vi "Lamp Name.vi"(7 "DB Data":variant[][](array[variant])) -> (1 "Led Name":string[](array[string]), 3 "Model Name":string)   [LabVIEW 2015]
uses:
  <vilib>/addons/database/_DB Variant To Data/Database Variant To Data.xnode
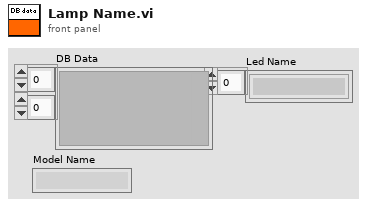
[diagram p1: front panel]
types:
  T1 = cluster{"Model Name":string, "Power Min":dbl, "Power Max":dbl, "Current Min":dbl, "Current Max":dbl, "Sleep Min ":dbl, "Sleep Max":dbl, "R-L Min":dbl, "R-L Max":dbl, "L-R Min":dbl, "L-R Max":dbl, "N-L Min":dbl, "N-L Max":dbl, "N-D Min":dbl, "N-D Max":dbl, "D-N Min":dbl, "D-N Max":dbl, "M-D Min":dbl, "M-D Max":dbl, "D-M Min":dbl, "D-M Max":dbl, "M-M+ Min":dbl, "M-M+ Max":dbl, "M-M- Min":dbl, "M-M- Max":dbl, "Part No":string, "Identify No":string, "Company Name":string, "Led_selection":u32, "LED1":string, "LED2":string, "LED3":string, "LED4":string}
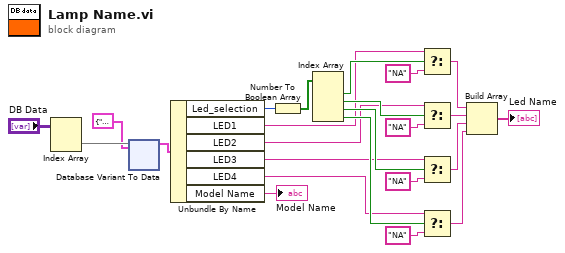
[diagram p0: block diagram]
diagram:
  n1 = Index Array(array="DB Data") -> (element=w10:variant[])  [unwired: 2 in]
  n2 = xnode "Database Variant To Data"("database variant"=w10, "type"=T1 {"Model Name"="", "Power Min"=0.0, "Power Max"=0.0, "Current Min"=0.0, "Current Max"=0.0, "Sleep Min "=0.0, "Sleep Max"=0.0, "R-L Min"=0.0, "R-L Max"=0.0, "L-R Min"=0.0, "L-R Max"=0.0, "N-L Min"=0.0, "N-L Max"=0.0, "N-D Min"=0.0, "N-D Max"=0.0, "D-N Min"=0.0, "D-N Max"=0.0, "M-D Min"=0.0, "M-D Max"=0.0, "D-M Min"=0.0, "D-M Max"=0.0, "M-M+ Min"=0.0, "M-M+ Max"=0.0, "M-M- Min"=0.0, "M-M- Max"=0.0, "Part No"="", "Identify No"="", "Company Name"="", "Led_selection"=0, "LED1"="", "LED2"="", "LED3"="", "LED4"=""} ("Read 2")) -> ("data"=w9:T1)  [unwired: 1 in, 1 out]
  n3 = Unbundle By Name(w9) -> ("Led_selection"=w6:u32, "LED1"=w5:string, "LED2"=w4:string, "LED3"=w3:string, "LED4"=w2:string, "Model Name"=→"Model Name":string)
  n4 = Number To Boolean Array(number=w6) -> (Boolean array=w16:bool[])
  n5 = Index Array(array=w16) -> (element #1=w17:bool, element #2=w20:bool, element #3=w22:bool, element #4=w24:bool)  [unwired: 4 in]
  n6 = Select(t=w5, s=w17, f="NA") -> (s? t:f=w15:string)
  n7 = Select(t=w4, s=w20, f="NA") -> (s? t:f=w14:string)
  n8 = Select(t=w3, s=w22, f="NA") -> (s? t:f=w13:string)
  n9 = Select(t=w2, s=w24, f="NA") -> (s? t:f=w12:string)
  n10 = Build Array(w15, w14, w13, w12) -> (→"Led Name":string[])
